vi "SPARK Configure Closed Loop Gains.vi"(6 "Closed Loop Slot (0)":T1 items=["Slot 0", "Slot 1", "Slot 2", "Slot 3"], 7 "Allowed Closed Loop Error":dbl=nan, 8 "error in":errorcluster, 9 "Feed Forward Gains":T2={"kV"=nan, "kS"=nan, "kA"=nan, "kG"=nan, "kCos"=nan, "kCosRatio"=nan}, 10 "PID Gains":T3={"kP"=nan, "kI"=nan, "kD"=nan}, 11 "MotorControlDeviceRef in":T4={"DeviceStatus"={"status"=FALSE, "code"=0, "source"=""}, "Type"=enum."PWM", "PWM"={"PWM Channel"=enum."Invalid", "DeadBand"={"Name"="", "maxPositivePwm"=0, "minPositivePwm"=0, "centerPwm"=0, "maxNegativePwm"=0, "minNegativePwm"=0, "angularRange"=0}}, "CAN"={"Device Number"=0, "SetOutput VI Ref"=variant(refnum<vi> refnum), "GetOutput VI Ref"=variant(refnum<vi> refnum), "Enable VI Ref"=variant(refnum<vi> refnum), "Disable VI Ref"=variant(refnum<vi> refnum), "Data"=variant}, "Invert"=FALSE, "DIO PWM"={"PWM \"Enable\" Channel"=enum."Invalid", "DIOChannel"=enum."Invalid", "PWM Rate"=0.0}}) -> (0 "error out":errorcluster, 3 "MotorControlDeviceRef out":T4={"DeviceStatus"={"status"=FALSE, "code"=0, "source"=""}, "Type"=enum."PWM", "PWM"={"PWM Channel"=enum."Invalid", "DeadBand"={"Name"="", "maxPositivePwm"=0, "minPositivePwm"=0, "centerPwm"=0, "maxNegativePwm"=0, "minNegativePwm"=0, "angularRange"=0}}, "CAN"={"Device Number"=0, "SetOutput VI Ref"=variant(refnum<vi> refnum), "GetOutput VI Ref"=variant(refnum<vi> refnum), "Enable VI Ref"=variant(refnum<vi> refnum), "Disable VI Ref"=variant(refnum<vi> refnum), "Data"=variant}, "Invert"=FALSE, "DIO PWM"={"PWM \"Enable\" Channel"=enum."Invalid", "DIOChannel"=enum."Invalid", "PWM Rate"=0.0}})   [LabVIEW 2023]
doc: "Configure the PID and feed forward gains for the closed loop controller of the SPARK."
uses:
  <vilib>/Rock Robotics/WPI/MotorControl/WPI_MotorControlDeviceRef.ctl
  <vilib>/Rock Robotics/WPI/MotorControl/WPI_MotorControlType.ctl
  <vilib>/Rock Robotics/SystemInterfaces/DIO/FPGA_DIOPWMChannel.ctl
  <vilib>/Rock Robotics/WPI/PWM/WPI_PWMDeadband.ctl
  <vilib>/Rock Robotics/SystemInterfaces/DIO/FPGA_DIOChannel.ctl
  Typedef/SPARK PID Gains.ctl
  Typedef/SPARK Feed Forward Gains.ctl
  Typedef/SPARK Closed Loop Slot.ctl
  Typedef/SPARK Parameter ID.ctl
  Private/SPARK/SPARK Set Parameter Float.vi
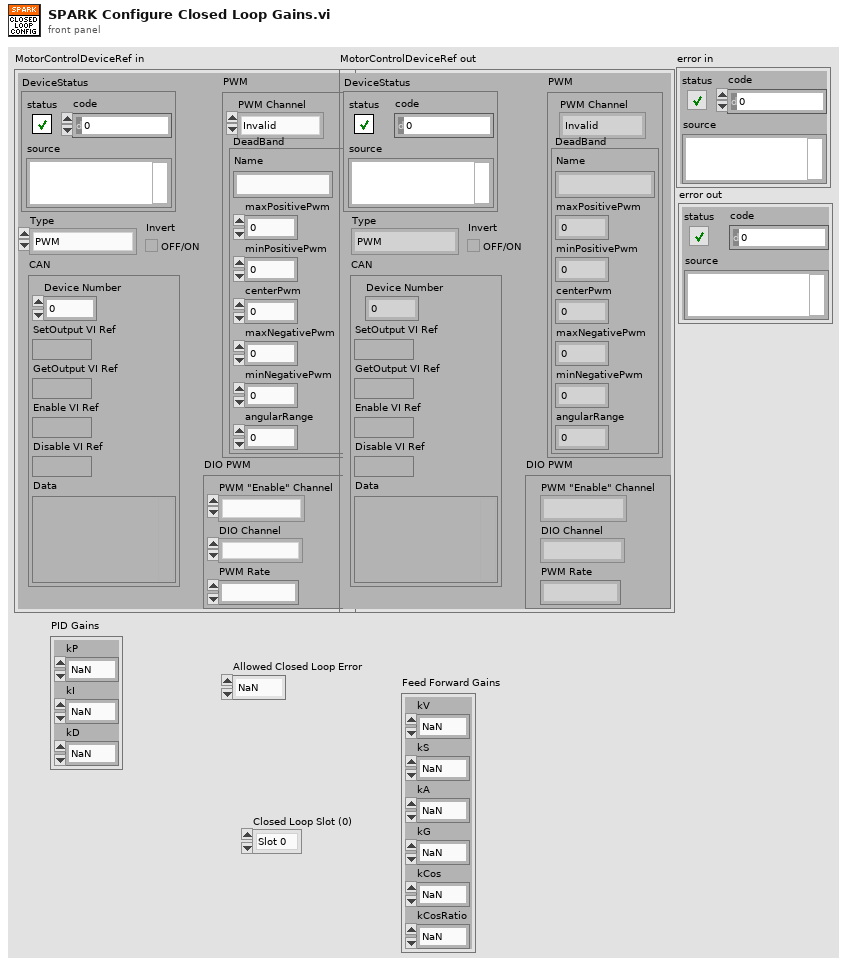
[diagram p1: front panel]
types:
  T1 = typedef "SPARK Closed Loop Slot.ctl" = u16
  T2 = typedef "SPARK Feed Forward Gains.ctl" = cluster{"kV":dbl, "kS":dbl, "kA":dbl, "kG":dbl, "kCos":dbl, "kCosRatio":dbl}
  T3 = typedef "SPARK PID Gains.ctl" = cluster{"kP":dbl, "kI":dbl, "kD":dbl}
  T4 = typedef "WPI_MotorControlDeviceRef.ctl" = cluster{"DeviceStatus":errorcluster, "Type":T5, "PWM":cluster{"PWM Channel":T6, "DeadBand":T7}, "CAN":cluster{"Device Number":u8, "SetOutput VI Ref":variant, "GetOutput VI Ref":variant, "Enable VI Ref":variant, "Disable VI Ref":variant, "Data":variant}, "Invert":bool, "DIO PWM":cluster{"PWM \"Enable\" Channel":T6, "DIOChannel":T8, "PWM Rate":dbl}}
  T5 = typedef "WPI_MotorControlType.ctl" = enum16{"PWM", "CAN", "DIO PWM"}
  T6 = typedef "FPGA_DIOPWMChannel.ctl" = enum8{"PWM 0", "PWM 1", "PWM 2", "PWM 3", "PWM 4", "PWM 5", "PWM 6", "PWM 7", "PWM 8", "PWM 9", "PWM MXP 0", "PWM MXP 1", "PWM MXP 2", "PWM MXP 3", "PWM MXP 4", "PWM MXP 5", "PWM MXP 6", "PWM MXP 7", "PWM MXP 8", "PWM MXP 9", "Invalid"}
  T7 = typedef "WPI_PWMDeadband.ctl" = cluster{"Name":string, "maxPositivePwm":i32, "minPositivePwm":i32, "centerPwm":i32, "maxNegativePwm":i32, "minNegativePwm":i32, "angularRange":u16}
  T8 = typedef "FPGA_DIOChannel.ctl" = enum8{"DIO 0", "DIO 1", "DIO 2", "DIO 3", "DIO 4", "DIO 5", "DIO 6", "DIO 7", "DIO 8", "DIO 9", "DIO MXP 0", "DIO MXP 1", "DIO MXP 2", "DIO MXP 3", "DIO MXP 4", "DIO MXP 5", "DIO MXP 6", "DIO MXP 7", "DIO MXP 8", "DIO MXP 9", "DIO MXP 10", "DIO MXP 11", "DIO MXP 12", "DIO MXP 13", "DIO MXP 14", "DIO MXP 15", "SPI Port CS1", "SPI Port CS2", "SPI Port CS3", "SPI Port MISO", "SPI Port MOSI", "Invalid"}
  T9 = typedef "SPARK Parameter ID.ctl" = enum16{"kCanID", "kInputMode", "kMotorType", "kCommAdvance", "kSensorType", "kCtrlType", "kIdleMode", "kInputDeadband", "kLegacyFeedbackSensorPID0", "kClosedLoopControlSensor", "kPolePairs", "kCurrentChop", "kCurrentChopCycles", "kP_0", "kI_0", "kD_0", "kV_0", "kIZone_0", "kDFilter_0", "kOutputMin_0", "kOutputMax_0", "kP_1", "kI_1", "kD_1", "kV_1", "kIZone_1", "kDFilter_1", "kOutputMin_1", "kOutputMax_1", "kP_2", "kI_2", "kD_2", "kV_2", "kIZone_2", "kDFilter_2", "kOutputMin_2", "kOutputMax_2", "kP_3", "kI_3", "kD_3", "kV_3", "kIZone_3", "kDFilter_3", "kOutputMin_3", "kOutputMax_3", "kInverted", "kOutputRatio", "kSerialNumberLow", "kSerialNumberMid", "kSerialNumberHigh", "kLimitSwitchFwdPolarity", "kLimitSwitchRevPolarity", "kHardLimitFwdEn", "kHardLimitRevEn", "kSoftLimitFwdEn", "kSoftLimitRevEn", "kRampRate", "kFollowerID", "kFollowerConfig", "kSmartCurrentStallLimit", "kSmartCurrentFreeLimit", "kSmartCurrentConfig", "kSmartCurrentReserved", "kMotorKv", "kMotorR", "kMotorL", "kMotorRsvd1", "kMotorRsvd2", "kMotorRsvd3", "kEncoderCountsPerRev", "kEncoderAverageDepth", "kEncoderSampleDelta", "kEncoderInverted", "kEncoderRsvd1", "kClosedLoopVoltageMode", "kCompensatedNominalVoltage", "kSmartMotionMaxVelocity_0", "kSmartMotionMaxAccel_0", "kSmartMotionMinVelOutput_0", "kSmartMotionAllowedClosedLoopError_0", "kSmartMotionAccelStrategy_0", "kSmartMotionMaxVelocity_1", "kSmartMotionMaxAccel_1", "kSmartMotionMinVelOutput_1", "kSmartMotionAllowedClosedLoopError_1", "kSmartMotionAccelStrategy_1", "kSmartMotionMaxVelocity_2", "kSmartMotionMaxAccel_2", "kSmartMotionMinVelOutput_2", "kSmartMotionAllowedClosedLoopError_2", "kSmartMotionAccelStrategy_2", "kSmartMotionMaxVelocity_3", "kSmartMotionMaxAccel_3", "kSmartMotionMinVelOutput_3", "kSmartMotionAllowedClosedLoopError_3", "kSmartMotionAccelStrategy_3", "kIMaxAccum_0", "kAllowedClosedLoopError_0", "kSlot3Placeholder2_0", "kSlot3Placeholder3_0", "kIMaxAccum_1", "kAllowedClosedLoopError_1", "kSlot3Placeholder2_1", "kSlot3Placeholder3_1", "kIMaxAccum_2", "kAllowedClosedLoopError_2", "kSlot3Placeholder2_2", "kSlot3Placeholder3_2", "kIMaxAccum_3", "kAllowedClosedLoopError_3", "kSlot3Placeholder2_3", "kSlot3Placeholder3_3", "kPositionConversionFactor", "kVelocityConversionFactor", "kClosedLoopRampRate", "kSoftLimitFwd", "kSoftLimitRev", "kSoftLimitRsvd0", "kSoftLimitRsvd1", "kAnalogPositionConversion", "kAnalogVelocityConversion", "kAnalogAverageDepth", "kAnalogSensorMode", "kAnalogInverted", "kAnalogSampleDelta", "kAnalogRsvd0", "kAnalogRsvd1", "kDataPortConfig", "kAltEncoderCountsPerRev", "kAltEncoderAverageDepth", "kAltEncoderSampleDelta", "kAltEncoderInverted", "kAltEncoderPositionConversion", "kAltEncoderVelocityConversion", "kAltEncoderRsvd0", "kAltEncoderRsvd1", "kHallSensorSampleRate", "kHallSensorAverageDepth", "kNumParameters", "kDutyCyclePositionFactor", "kDutyCycleVelocityFactor", "kDutyCycleInverted", "kDutyCycleSensorMode", "kDutyCycleAverageDepth", "kDutyCycleSampleDelta", "kDutyCycleOffsetv1p6p2", "kDutyCycleRsvd0", "kDutyCycleRsvd1", "kDutyCycleRsvd2", "kPositionPIDWrapEnable", "kPositionPIDMinInput", "kPositionPIDMaxInput", "kDutyCycleZeroCentered", "kDutyCyclePrescalar", "kDutyCycleOffset", "kProductId", "kDeviceMajorVersion", "kDeviceMinorVersion", "kStatus0Period", "kStatus1Period", "kStatus2Period", "kStatus3Period", "kStatus4Period", "kStatus5Period", "kStatus6Period", "kStatus7Period", "kMAXMotionCruiseVelocity_0", "kMAXMotionMaxAccel_0", "kMAXMotionMaxJerk_0", "kMAXMotionAllowedProfileError_0", "kMAXMotionPositionMode_0", "kMAXMotionCruiseVelocity_1", "kMAXMotionMaxAccel_1", "kMAXMotionMaxJerk_1", "kMAXMotionAllowedProfileError_1", "kMAXMotionPositionMode_1", "kMAXMotionCruiseVelocity_2", "kMAXMotionMaxAccel_2", "kMAXMotionMaxJerk_2", "kMAXMotionAllowedProfileError_2", "kMAXMotionPositionMode_2", "kMAXMotionCruiseVelocity_3", "kMAXMotionMaxAccel_3", "kMAXMotionMaxJerk_3", "kMAXMotionAllowedProfileError_3", "kMAXMotionPositionMode_3", "kForceEnableStatus0", "kForceEnableStatus1", "kForceEnableStatus2", "kForceEnableStatus3", "kForceEnableStatus4", "kForceEnableStatus5", "kForceEnableStatus6", "kForceEnableStatus7", "kFollowerModeLeaderId", "kFollowerModeIsInverted", "kDutyCycleEncoderStartPulseUs", "kDutyCycleEncoderEndPulseUs", "kParamTableVersion", "kStatus8Period", "kForceEnableStatus8", "kLimitSwitchPositionSensor", "kLimitSwitchForwardPosition", "kLimitSwitchReversePosition", "kS_0", "kA_0", "kG_0", "kCos_0", "kCosRatio_0", "kS_1", "kA_1", "kG_1", "kCos_1", "kCosRatio_1", "kS_2", "kA_2", "kG_2", "kCos_2", "kCosRatio_2", "kS_3", "kA_3", "kG_3", "kCos_3", "kCosRatio_3", "kStatus9Period", "kForceEnableStatus9"}
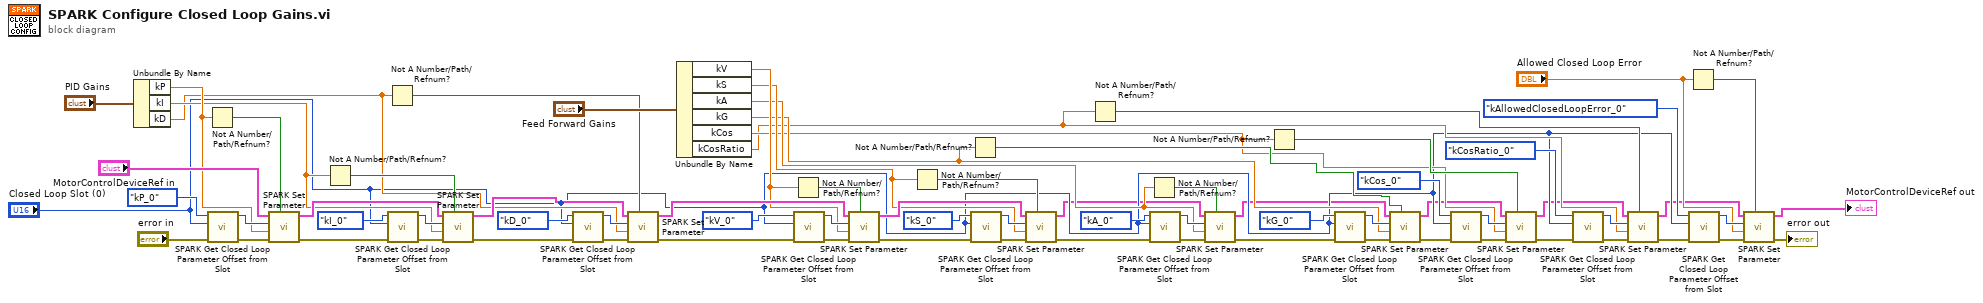
[diagram p0: block diagram]
diagram:
  n1 = Unbundle By Name("PID Gains") -> ("kP"=w51:dbl, "kI"=w49:dbl, "kD"=w47:dbl)
  n2 = Not A Number/Path/Refnum?(number/path/refnum=w51) -> (NaN/Path/Refnum?=w50:bool)
  n3 = call "SPARK Get Closed Loop Parameter Offset from Slot.vi"("error in (no error)"="error in", "Closed Loop Slot"="Closed Loop Slot (0)", "Parameter ID in"=SPARK_Parameter_ID."kP_0") -> ("error out"=w66:errorcluster, "Parameter ID out"=w71:T9)  [unwired: 7 in]
  n4 = call-poly "SPARK Set Parameter.vi"("Ignore"=w50, "error in (no error)"=w66, "single precision float"=w51, "Parameter ID"=w71, "MotorControlDeviceRef"="MotorControlDeviceRef in") -> ("error out"=w65:errorcluster, "MotorControlDeviceRef"=w60:T4)  [unwired: 5 in]
  n5 = Not A Number/Path/Refnum?(number/path/refnum=w49) -> (NaN/Path/Refnum?=w48:bool)
  n6 = Not A Number/Path/Refnum?(number/path/refnum=w47) -> (NaN/Path/Refnum?=w46:bool)
  n7 = call "SPARK Get Closed Loop Parameter Offset from Slot.vi"("error in (no error)"=w65, "Closed Loop Slot"="Closed Loop Slot (0)", "Parameter ID in"=SPARK_Parameter_ID."kI_0") -> ("error out"=w64:errorcluster, "Parameter ID out"=w70:T9)  [unwired: 7 in]
  n8 = call-poly "SPARK Set Parameter.vi"("Ignore"=w48, "error in (no error)"=w64, "single precision float"=w49, "Parameter ID"=w70, "MotorControlDeviceRef"=w60) -> ("error out"=w63:errorcluster, "MotorControlDeviceRef"=w61:T4)  [unwired: 5 in]
  n9 = call "SPARK Get Closed Loop Parameter Offset from Slot.vi"("error in (no error)"=w63, "Closed Loop Slot"="Closed Loop Slot (0)", "Parameter ID in"=SPARK_Parameter_ID."kD_0") -> ("error out"=w62:errorcluster, "Parameter ID out"=w69:T9)  [unwired: 7 in]
  n10 = call-poly "SPARK Set Parameter.vi"("Ignore"=w46, "error in (no error)"=w62, "single precision float"=w47, "Parameter ID"=w69, "MotorControlDeviceRef"=w61) -> ("error out"=w56:errorcluster, "MotorControlDeviceRef"=w59:T4)  [unwired: 5 in]
  n11 = Unbundle By Name("Feed Forward Gains") -> ("kV"=w53:dbl, "kS"=w32:dbl, "kA"=w15:dbl, "kG"=w14:dbl, "kCos"=w13:dbl, "kCosRatio"=w12:dbl)
  n12 = Not A Number/Path/Refnum?(number/path/refnum=w53) -> (NaN/Path/Refnum?=w52:bool)
  n13 = call "SPARK Get Closed Loop Parameter Offset from Slot.vi"("error in (no error)"=w56, "Closed Loop Slot"="Closed Loop Slot (0)", "Parameter ID in"=SPARK_Parameter_ID."kV_0") -> ("error out"=w55:errorcluster, "Parameter ID out"=w58:T9)  [unwired: 7 in]
  n14 = call-poly "SPARK Set Parameter.vi"("Ignore"=w52, "error in (no error)"=w55, "single precision float"=w53, "Parameter ID"=w58, "MotorControlDeviceRef"=w59) -> ("error out"=w34:errorcluster, "MotorControlDeviceRef"=w33:T4)  [unwired: 5 in]
  n15 = Not A Number/Path/Refnum?(number/path/refnum=w32) -> (NaN/Path/Refnum?=w38:bool)
  n16 = Not A Number/Path/Refnum?(number/path/refnum=w14) -> (NaN/Path/Refnum?=w27:bool)
  n17 = call "SPARK Get Closed Loop Parameter Offset from Slot.vi"("error in (no error)"=w34, "Closed Loop Slot"="Closed Loop Slot (0)", "Parameter ID in"=SPARK_Parameter_ID."kS_0") -> ("error out"=w37:errorcluster, "Parameter ID out"=w35:T9)  [unwired: 7 in]
  n18 = call-poly "SPARK Set Parameter.vi"("Ignore"=w38, "error in (no error)"=w37, "single precision float"=w32, "Parameter ID"=w35, "MotorControlDeviceRef"=w33) -> ("error out"=w10:errorcluster, "MotorControlDeviceRef"=w1:T4)  [unwired: 5 in]
  n19 = Not A Number/Path/Refnum?(number/path/refnum=w12) -> (NaN/Path/Refnum?=w19:bool)
  n20 = Not A Number/Path/Refnum?(number/path/refnum=w15) -> (NaN/Path/Refnum?=w28:bool)
  n21 = call "SPARK Get Closed Loop Parameter Offset from Slot.vi"("error in (no error)"=w10, "Closed Loop Slot"="Closed Loop Slot (0)", "Parameter ID in"=SPARK_Parameter_ID."kA_0") -> ("error out"=w29:errorcluster, "Parameter ID out"=w31:T9)  [unwired: 7 in]
  n22 = call-poly "SPARK Set Parameter.vi"("Ignore"=w28, "error in (no error)"=w29, "single precision float"=w15, "Parameter ID"=w31, "MotorControlDeviceRef"=w1) -> ("error out"=w9:errorcluster, "MotorControlDeviceRef"=w2:T4)  [unwired: 5 in]
  n23 = Not A Number/Path/Refnum?(number/path/refnum=w13) -> (NaN/Path/Refnum?=w20:bool)
  n24 = call "SPARK Get Closed Loop Parameter Offset from Slot.vi"("error in (no error)"=w9, "Closed Loop Slot"="Closed Loop Slot (0)", "Parameter ID in"=SPARK_Parameter_ID."kG_0") -> ("error out"=w26:errorcluster, "Parameter ID out"=w24:T9)  [unwired: 7 in]
  n25 = call-poly "SPARK Set Parameter.vi"("Ignore"=w27, "error in (no error)"=w26, "single precision float"=w14, "Parameter ID"=w24, "MotorControlDeviceRef"=w2) -> ("error out"=w8:errorcluster, "MotorControlDeviceRef"=w3:T4)  [unwired: 5 in]
  n26 = call "SPARK Get Closed Loop Parameter Offset from Slot.vi"("error in (no error)"=w8, "Closed Loop Slot"="Closed Loop Slot (0)", "Parameter ID in"=SPARK_Parameter_ID."kCos_0") -> ("error out"=w21:errorcluster, "Parameter ID out"=w23:T9)  [unwired: 7 in]
  n27 = call-poly "SPARK Set Parameter.vi"("Ignore"=w20, "error in (no error)"=w21, "single precision float"=w13, "Parameter ID"=w23, "MotorControlDeviceRef"=w3) -> ("error out"=w7:errorcluster, "MotorControlDeviceRef"=w6:T4)  [unwired: 5 in]
  n28 = call "SPARK Get Closed Loop Parameter Offset from Slot.vi"("error in (no error)"=w7, "Closed Loop Slot"="Closed Loop Slot (0)", "Parameter ID in"=SPARK_Parameter_ID."kCosRatio_0") -> ("error out"=w18:errorcluster, "Parameter ID out"=w16:T9)  [unwired: 7 in]
  n29 = call-poly "SPARK Set Parameter.vi"("Ignore"=w19, "error in (no error)"=w18, "single precision float"=w12, "Parameter ID"=w16, "MotorControlDeviceRef"=w6) -> ("error out"=w4:errorcluster, "MotorControlDeviceRef"=w5:T4)  [unwired: 5 in]
  n30 = Not A Number/Path/Refnum?(number/path/refnum="Allowed Closed Loop Error") -> (NaN/Path/Refnum?=w39:bool)
  n31 = call "SPARK Get Closed Loop Parameter Offset from Slot.vi"("error in (no error)"=w4, "Closed Loop Slot"="Closed Loop Slot (0)", "Parameter ID in"=SPARK_Parameter_ID."kAllowedClosedLoopError_0") -> ("error out"=w44:errorcluster, "Parameter ID out"=w43:T9)  [unwired: 7 in]
  n32 = call-poly "SPARK Set Parameter.vi"("Ignore"=w39, "error in (no error)"=w44, "single precision float"="Allowed Closed Loop Error", "Parameter ID"=w43, "MotorControlDeviceRef"=w5) -> ("error out"=→"error out":errorcluster, "MotorControlDeviceRef"=→"MotorControlDeviceRef out":T4)  [unwired: 5 in]
